vi "Collect and Merge All Active ActorRef.vi"(8 "Error In":errorcluster, 11 "Core In":refnum<class "Core.lvclass">) -> (0 "Error Out":errorcluster, 3 "Core Out":refnum<class "Core.lvclass">)   [LabVIEW 2019, in "Core.lvlib" / "Core.lvclass"]
uses:
  Core.lvclass
  ModuleAbstract/ModuleAbstract.lvclass
  C:/Projekty/_Wewnetrzne/PC_ActorFramework/07_Program/LABVIEW/02_Source/Modules/ModuleAbstract/ModuleAbstract.lvclass
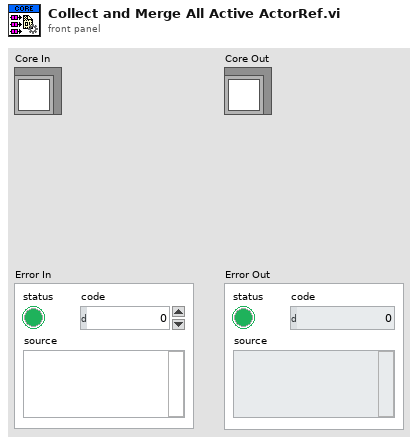
[diagram p1: front panel]
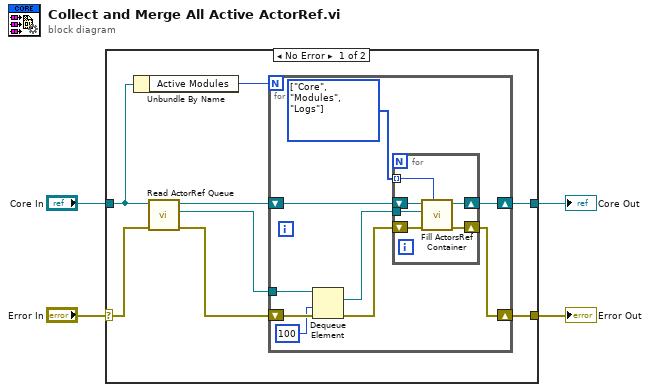
[diagram p0: block diagram]
diagram:
  n1 = case shown="No Error" "Error In" {
    selector: "Error In" -> [w8 w29]
    tunnel: [w12 w28] -> w4
    tunnel: [w11 w29] -> w3
    tunnel: "Core In" -> [w6 w28]
    frame No Error {
      n2 = Unbundle By Name(w6) -> ("Active Modules"=w5:i32)
      n3 = call "Read ActorRef Queue.vi"("error in (no error)"=w8, "ModuleAbstract in"=w6) -> ("error out"=w7:errorcluster, "ActorRef Queue"=w9:refnum<queue>, "ModuleAbstract out"=w10:refnum<class "Core.lvclass">)  [unwired: 7 in]
      n4 = for {
        N: w5 -> [_]
        shift-right: [w15] -> w11
        shift-left: w7 -> [w21]
        shift-right: [w16] -> w12
        shift-left: w10 -> [w17]
        tunnel: w9 -> [w14]
        w13 = enum16{"Core", "Modules", "Logs"}[] [enum."Core", enum."Modules", enum."Logs"] items=["Core", "Modules", "Logs"] ("Mode")
        n5 = Dequeue Element(queue=w14, timeout in ms (-1)=100, error in (no error)=w21) -> (element=w18:refnum<class "ActorRefContainer.lvclass">, error out=w19:errorcluster)  [unwired: 2 out]
        n6 = for {
          tunnel: w18 -> [w26]
          shift-right: [w23] -> w15
          shift-left: w19 -> [w27]
          shift-right: [w24] -> w16
          shift-left: w17 -> [w25]
          tunnel: w13 -> [w22] mode=indexing
          n7 = call "Fill ActorsRef Container.vi"("Mode"=w22, "error in (no error)"=w27, "Ref Data Object"=w26, "Core In"=w25) -> ("error out"=w23:errorcluster, "Core Out"=w24:refnum<class "Core.lvclass">)  [unwired: 6 in]
        }
      }
    }
    frame Error {
    }
  }
  "Core Out" <- w4
  "Error Out" <- w3
